vi "PYTHON Set Data__ogtk.vi"   [LabVIEW 2012]
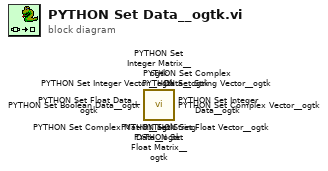
[diagram p0: block diagram]
diagram:
  n1 = call <userlib>:"PYTHON Set String Data__ogtk.vi"() -> ()  [unwired: 6 in, 2 out]
  n2 = call <userlib>:"PYTHON Set Complex Data__ogtk.vi"() -> ()  [unwired: 6 in, 2 out]
  n3 = call <userlib>:"PYTHON Set Float Data__ogtk.vi"() -> ()  [unwired: 6 in, 2 out]
  n4 = call <userlib>:"PYTHON Set Integer Data__ogtk.vi"() -> ()  [unwired: 6 in, 2 out]
  n5 = call <userlib>:"PYTHON Set Integer Vector__ogtk.vi"() -> ()  [unwired: 6 in, 2 out]
  n6 = call <userlib>:"PYTHON Set Integer Matrix__ogtk.vi"() -> ()  [unwired: 6 in, 2 out]
  n7 = call <userlib>:"PYTHON Set Float Vector__ogtk.vi"() -> ()  [unwired: 6 in, 2 out]
  n8 = call <userlib>:"PYTHON Set Float Matrix__ogtk.vi"() -> ()  [unwired: 6 in, 2 out]
  n9 = call <userlib>:"PYTHON Set Complex Vector__ogtk.vi"() -> ()  [unwired: 6 in, 2 out]
  n10 = call <userlib>:"PYTHON Set Complex Matrix__ogtk.vi"() -> ()  [unwired: 6 in, 2 out]
  n11 = call <userlib>:"PYTHON Set Boolean Data__ogtk.vi"() -> ()  [unwired: 6 in, 2 out]
  n12 = call <userlib>:"PYTHON Set String Vector__ogtk.vi"() -> ()  [unwired: 6 in, 2 out]
